vi "Read Alarm Status.vi"(8 "error in":errorcluster, 10 "alarm status in":T1, 11 "PV Data in":refnum<class "PV Data.lvclass">) -> (0 "error out":errorcluster, 1 "has alarm status?":bool, 2 "alarm status out":T1, 3 "PV Data out":refnum<class "PV Data.lvclass">)   [LabVIEW 2020, in "PV Access.lvlib" / "PV Data.lvlib" / "PV Data.lvclass"]
uses:
  PV Data.lvclass
  PV Access.lvlib
  <vilib>/addons/Tools/Unicode/UTF8 Tools.lvlib
  Alarm.ctl
  PV Data.lvlib
  Alarm Severity.ctl
  Alarm Status.ctl
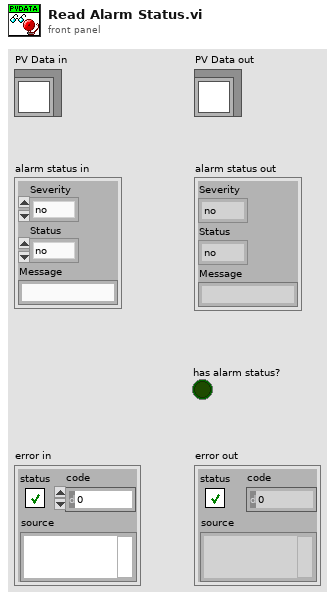
[diagram p1: front panel]
types:
  T1 = typedef "PV Access.lvlib/PV Data.lvlib/Alarm.ctl" = cluster{"Severity":T2, "Status":T3, "Message":string}
  T2 = typedef "PV Access.lvlib/PV Data.lvlib/Alarm Severity.ctl" = enum32{"no", "minor", "major", "record", "invalid", "undefined", ""}
  T3 = typedef "PV Access.lvlib/PV Data.lvlib/Alarm Status.ctl" = enum32{"no", "device", "driver", "record", "db", "conf", "undefined", "client"}
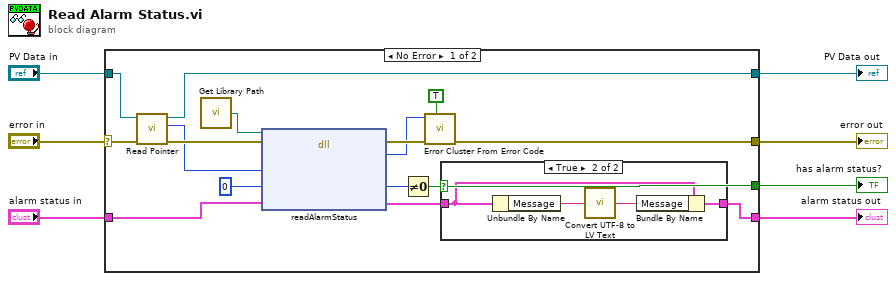
[diagram p0: block diagram]
diagram:
  n1 = case shown="No Error" "error in" {
    selector: "error in" -> [w18 w31]
    tunnel: [w19 w31] -> w7
    tunnel: "PV Data in" -> [w16 w30]
    tunnel: [w14 w30] -> w4
    tunnel: "alarm status in" -> [w13 w29]
    tunnel: [w10 _] -> w3
    tunnel: [w8 w29] -> w1
    frame No Error {
      n2 = call-dynamic "Read Pointer.vi"("error in (no error)"=w18, "Pointer Base in"=w16) -> ("error out"=w17:errorcluster, "Pointer"=w15:i64, "Pointer Base out"=w14:refnum<class "PV Data.lvclass">)  [unwired: 7 in]
      n3 = call "Get Library Path.vi"() -> ("Path"=w23:path)  [unwired: 1 in]
      n4 = dll-call lib="?" fn="readAlarmStatus"(path in=w23, error in=w17, "value"=w15, "has alarm status?"=i16 0 ("has display metadata?"), "alarm status"=w13) -> (error out=w21:errorcluster, "err_code"=w20:i32, "has alarm status?"=w12:i16, "alarm status"=w9:T1)  [unwired: 2 in, 1 out]
      n5 = Not Equal To 0?(x=w12) -> (x != 0?=w10:bool)
      n6 = call <vilib>:"Error Cluster From Error Code.vi"("show call chain? (False)"=TRUE, "error in (no error)"=w21, "error code (0)"=w20) -> ("error out"=w19:errorcluster)  [unwired: 6 in]
      n7 = case shown="True" w10 {
        tunnel: w9 -> [w24 w27]
        tunnel: [w24 w25] -> w8
        frame False {
        }
        frame True {
          n8 = Unbundle By Name(w27) -> ("Message"=w28:string)
          n9 = call <vilib>:"Convert UTF-8 to LV Text.vi"("UTF-8 Text"=w28) -> ("LV Text"=w26:string)  [unwired: 13 in, 1 out]
          n10 = Bundle By Name(cluster=w27, "Message"=w26) -> (w25:T1)
        }
      }
    }
    frame Error {
    }
  }
  "error out" <- w7
  "PV Data out" <- w4
  "has alarm status?" <- w3
  "alarm status out" <- w1
